vi "testCANopen.vi"() -> ()   [LabVIEW 2024]
doc: "Tests CANopen (and possibly CANbus) nets exercising the CANopen.lvclass APIs."
uses:
  CANopen/Multiplexor.ctl
  CANopen/FunctionCode.ctl
  DSP402/DSP402.lvclass
  CANopen/CANopen.lvclass
  DSP402/DriveState.ctl
  DSP402/DriveMode.ctl
  HAL/HAL/Devices/CAN Interfaces/PCAN/PCAN.lvclass
  D:/git/HAL/HAL/Configurations/CFG Base/CFG Base.lvclass
  D:/git/HAL/HAL/Protocols/ICAN/ICAN.lvclass
  CANopen/CANopen.lvclass/CANopen.ctl
  types/threestateFlag.ctl
  canopen.lvlib
  HAL/HAL/Configurations/CFG Base/CFG Base.lvclass
panel:
  in  "CANopen":refnum<class "CANopen.lvclass">
  in  "DSP402":refnum<class "DSP402.lvclass">
  in  "Variant":variant=variant(u8[] [80, 0])
  in  "Tab Control":T1(tab)
  in  "NMT send":bool
  in  "Node ID (NMT)":u8=50 caption="Node ID"
  in  "Command specifier":u8(ring)=129 items=["Start remote node"=1, "Stop remote node"=2, "Enter pre-operational state"=128, "Reset node"=129, "Reset communication"=130]
  in  "SDO size":u8=2 caption="Bytes" format="%0d"
  in  "SDO read":bool
  in  "Multiplexor":T2={"Index"=4119, "Sub-index"=0} {"Sub-index" format="%02x"; "Index" format="%04x"}
  in  "SDO value":u32 caption="Value" format="%08x"
  in  "SDO write":bool
  in  "Node ID (SDO)":u8=50 caption="Node ID"
  in  "Remap TxPDO":bool
  in  "TxPDO map":cluster{"CobID":u32, "nBytes":u8}[](array[cluster])=[{"CobID"=434, "nBytes"=2}] {"CobID" format="%x"}
  out "Input image":bool[](array[boolean])
  in  "Remap RxPDO":bool
  in  "RxPDO map":cluster{"CobID":u32, "nBytes":u8}[](array[cluster])=[{"CobID"=562, "nBytes"=5}] {"CobID" format="%x"}
  in  "Output image":bool[](array[boolean])
  in  "Node ID (402)":u8 caption="Node ID"
  in  "State (402)":T3 caption="State"
  in  "Mode (402)":T4 caption="Mode" items=["Undefined"=0, "Profile Position Mode"=1, "Velocity Mode"=2, "Profile Velocity Mode"=3, "Torque Profile Mode"=4, "Homing Mode"=6, "Interpolated Position Mode"=7]
  in  "Position (402)":u32 caption="Position"
  in  "Speed (402)":i16=500 caption="Speed (RpM)"
  in  "Operation flags (402)":cluster{"ON":bool, "OFF":bool}[](array[cluster]) caption="Force bit 4, 5, 6 and Halt"
  in  "Acceleration (402)":u32=100 caption="Acc"
  in  "Deceleration (402)":u32=100 caption="Dec"
  in  "Get status (402)":bool
  in  "PDO unlink":bool
  in  "PDO link":bool
  in  "Node ID (link)":u8=50 caption="Node ID"
  in  "Function code (link)":T5=4 caption="Function code" items=["NMT", "SYNC", "TIME STAMP", "EMERGENCY", "PDO1 (tx)", "PDO1 (rx)", "PDO2 (tx)", "PDO2 (rx)", "PDO3 (tx)", "PDO3 (rx)", "PDO4 (tx)", "PDO4 (rx)", "SDO (tx)", "SDO (rx)", "NMT Error Control"]
  in  "Indices":cluster{"Communication":u32, "Mapping":u32}={"Communication"=6144, "Mapping"=6656} {"Mapping" format="%x"; "Communication" format="%x"}
  in  "Map":cluster{"Multiplexor":T2, "nBits":u8}[](array[cluster])=[{"Multiplexor"={"Index"=24832, "Sub-index"=1}, "nBits"=16}] {"Multiplexor"."Sub-index" format="%02x"; "Multiplexor"."Index" format="%04x"}
  in  "Heartbeat set":bool
  in  "Heartbeat table":T6(array[cluster]) {"Period" format="%#.3g"}
  in  "Raw send":bool
  in  "Data (raw)":u8[](array[numeric]) caption="Data" format="%02x"
  in  "Node ID (raw)":u8 caption="Node ID"
  in  "Function code (raw)":T5=1 items=["NMT", "SYNC", "TIME STAMP", "EMERGENCY", "PDO1 (tx)", "PDO1 (rx)", "PDO2 (tx)", "PDO2 (rx)", "PDO3 (tx)", "PDO3 (rx)", "PDO4 (tx)", "PDO4 (rx)", "SDO (tx)", "SDO (rx)", "NMT Error Control"]
  in  "Stop":bool
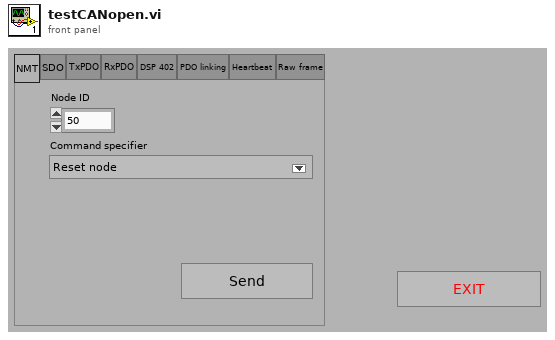
[diagram p1: front panel]
types:
  T1 = enum32{"NMT", "SDO", "TxPDO", "RxPDO", "DSP 402", "PDO linking", "Heartbeat", "Raw frame"}
  T2 = typedef "canopen.lvlib/CANopen.lvclass/Multiplexor.ctl" = cluster{"Index":u16, "Sub-index":u8}
  T3 = typedef "canopen.lvlib/DSP402.lvclass/DriveState.ctl" = enum16{"Start", "Not ready to switch on", "Switch on disabled", "Ready to switch on", "Switched on", "Operation enable", "Fault reaction active", "Fault", "Quick stop active"}
  T4 = typedef "canopen.lvlib/DSP402.lvclass/DriveMode.ctl" = i8
  T5 = typedef "canopen.lvlib/CANopen.lvclass/FunctionCode.ctl" = u8
  T6 = cluster{"Node ID":u8, "Period":dbl, "Set value":i16, "Value":i16}[]
  T7 = typedef "canopen.lvlib/threestateFlag.ctl" = i8
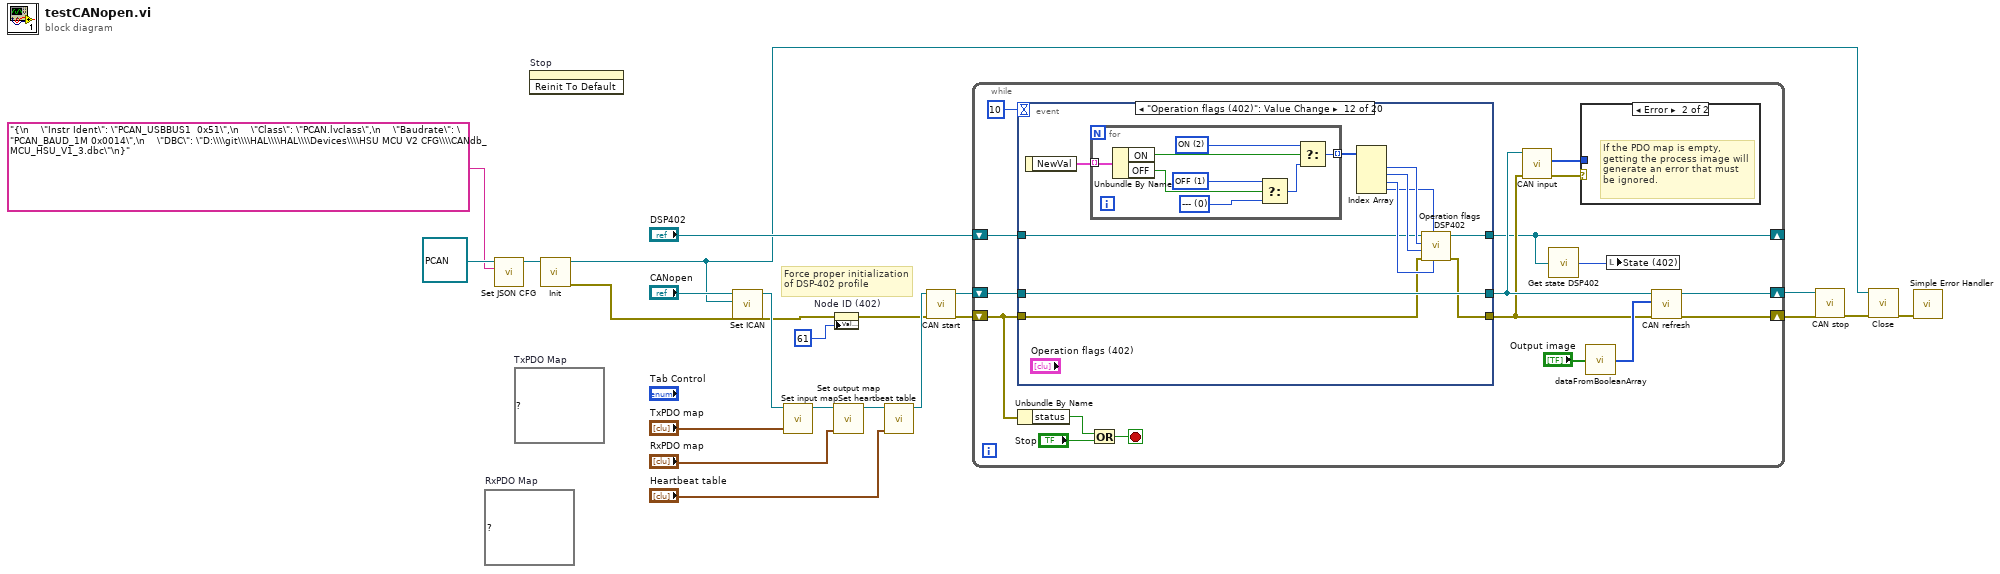
[diagram p0: block diagram]
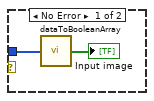
[diagram p2: hidden frame]
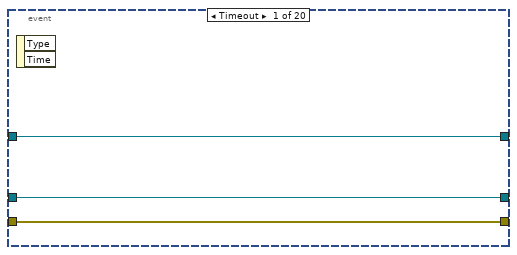
[diagram p3: hidden frame]
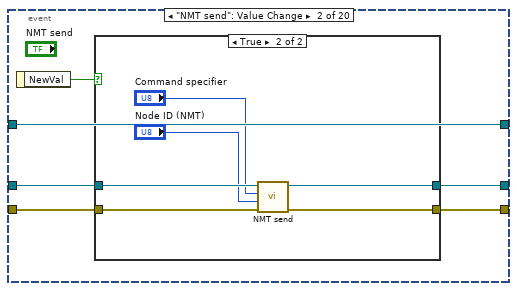
[diagram p4: hidden frame]
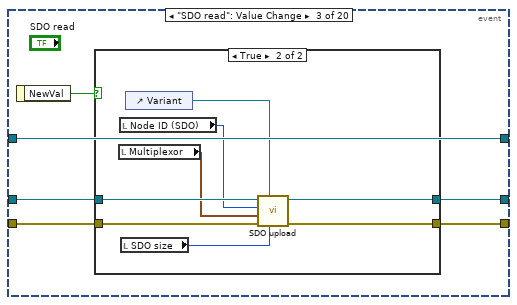
[diagram p6: hidden frame]
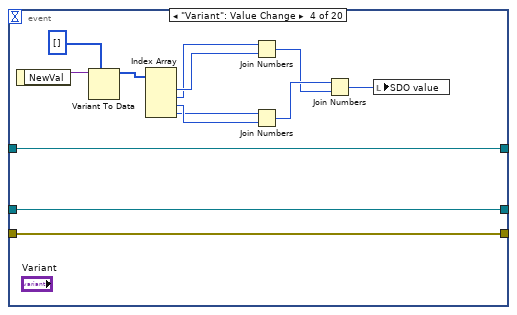
[diagram p8: hidden frame]
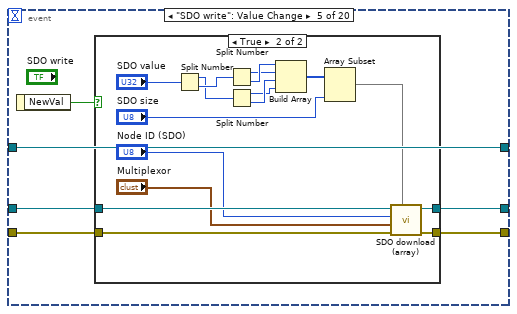
[diagram p9: hidden frame]
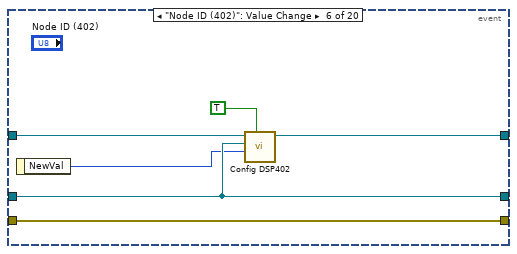
[diagram p11: hidden frame]
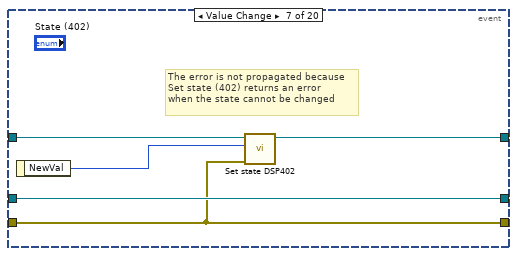
[diagram p12: hidden frame]
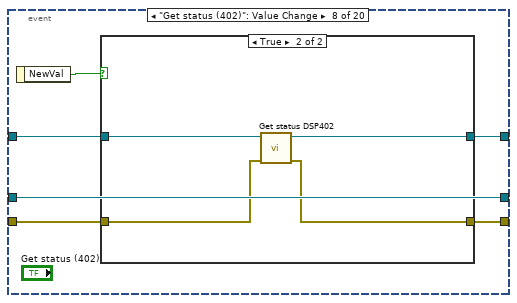
[diagram p13: hidden frame]
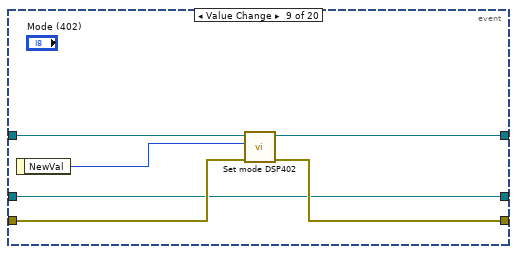
[diagram p15: hidden frame]
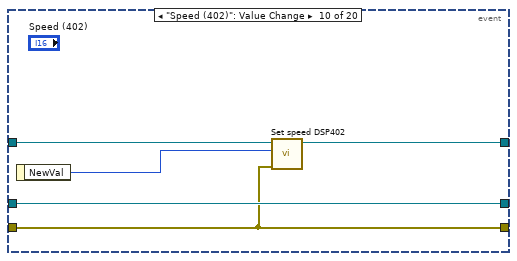
[diagram p16: hidden frame]
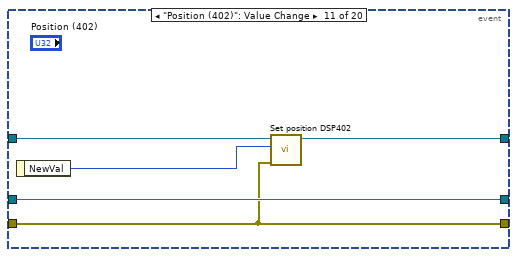
[diagram p17: hidden frame]
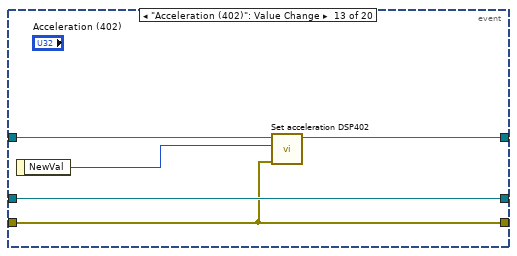
[diagram p18: hidden frame]
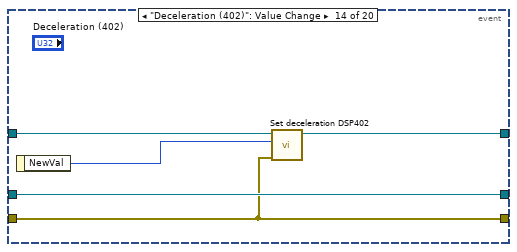
[diagram p19: hidden frame]
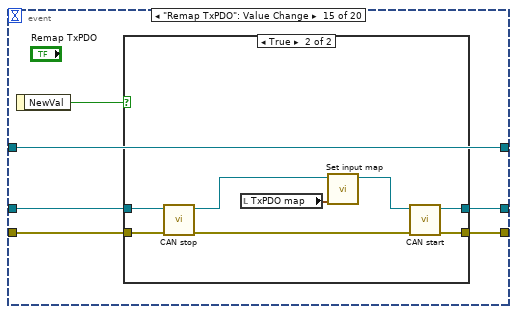
[diagram p20: hidden frame]
diagram:
  (unwired) map{u32, u32} {}  # RxPDO Map
  (unwired) map{u32, u32} {}  # TxPDO Map
  # "Force proper initialization\nof DSP-402 profile"
  n1 = call "Set JSON CFG.vi"("<JSON>CFG"="{\n    \"Instr Ident\": \"PCAN_USBBUS1  0x51\",\n    \"Class\": \"PCAN.lvclass\",\n    \"Baudrate\": \"PCAN_BAUD_1M 0x0014\",\n    \"DBC\": \"D:\\\\git\\\\HAL\\\\HAL\\\\Devices\\\\HSU MCU V2 CFG\\\\CANdb_MCU_HSU_V1_3.dbc\"\n}", "CFG Base in"=refnum<class "PCAN.lvclass"> refnum ("PCAN.lvclass")) -> ("CFG Base out"=w9:refnum<class "PCAN.lvclass">)  [unwired: 9 in]
  n2 = invoke on="Stop" class="Bool (strict)" method="Reinit To Default"() -> ()  [unwired: 3 in, 3 out]
  n3 = call-dynamic "Init.vi"("PCAN in"=w9) -> ("error out"=w1:errorcluster, "PCAN out"=w7:refnum<class "PCAN.lvclass">)  [unwired: 9 in]
  n4 = call "Set ICAN.vi"("ICAN"=w7, "CANopen in"="CANopen") -> ("CANopen out"=w2:refnum<class "CANopen.lvclass">)  [unwired: 9 in]
  n5 = call "Set input map.vi"("Map"="TxPDO map", "CANopen in"=w2) -> ("CANopen out"=w19:refnum<class "CANopen.lvclass">)  [unwired: 5 out]
  n6 = call "Set output map.vi"("Map"="RxPDO map", "CANopen in"=w19) -> ("CANopen out"=w17:refnum<class "CANopen.lvclass">)  [unwired: 5 out]
  n7 = property on="Node ID (402)" class="DigNum (strict)"(error in=w1, "Val(Sgnl)"=u8 61 ("Value (Signaling)")) -> (error out=w12:errorcluster)  [unwired: 1 in, 1 out]
  n8 = call "Set heartbeat table.vi"("Heartbeat table"="Heartbeat table", "CANopen in"=w17) -> ("CANopen out"=w15:refnum<class "CANopen.lvclass">)  [unwired: 1 in, 4 out]
  n9 = call "CAN start.vi"("error in (no error)"=w12, "CANopen in"=w15) -> ("error out"=w14:errorcluster, "CANopen out"=w20:refnum<class "CANopen.lvclass">)  [unwired: 4 out]
  n10 = while {
    shift-right: [w29] -> w5
    shift-left: w14 -> [w37]
    shift-right: [w28] -> w3
    shift-left: w20 -> [w39]
    shift-right: [w24] -> _
    shift-left: "DSP402" -> [w25]
    stop <- w36 stop-if-true
    n11 = event shown="[11] \"Operation flags (402)\": Value Change" {
      selector: _ -> [_ _ _ _ _ _ _ _ _ _ _ _ _ _ _ _ _ _ _ _]
      dyn-events: _ -> [_ _ _ _ _ _ _ _ _ _ _ _ _ _ _ _ _ _ _ _]
      timeout: 10 -> [_ _ _ _ _ _ _ _ _ _ _ _ _ _ _ _ _ _ _ _]
      tunnel: [w44 w50 w64 w87 w93 w115 w122 w123 w138 w145 w150 w160 w174 w179 w185 w201 w217 w229 w246 w262] -> w27
      tunnel: w39 -> [w44 w49 w63 w87 w92 w115 w122 w123 w138 w145 w150 w160 w174 w179 w184 w200 w216 w228 w245 w261]
      tunnel: [w43 w48 w62 w86 w91 w113 w118 w128 w139 w141 w146 w153 w170 w175 w183 w199 w215 w227 w244 w260] -> w26
      tunnel: w37 -> [w43 w47 w61 w86 w90 w113 w118 w127 w140 w141 w146 w154 w170 w175 w182 w198 w214 w226 w243 w259]
      tunnel: w25 -> [w42 w45 w59 w75 w88 w117 w120 w124 w136 w143 w149 w151 w172 w177 w180 w196 w212 w224 w241 w257]
      tunnel: [w42 w45 w59 w75 w88 w116 w119 w125 w135 w142 w148 w152 w171 w176 w180 w196 w212 w224 w241 w257] -> w24
      event Timeout {
        n12 = event-data() -> ()  [unwired: 3 out]
      }
      event "NMT send": Value Change {
        n13 = event-data() -> ("NewVal"=w46:bool)  [unwired: 1 out]
        n14 = case shown="True" w46 {
          tunnel: [w52 w55] -> w50
          tunnel: w49 -> [w52 w58]
          tunnel: [w51 w56] -> w48
          tunnel: w47 -> [w51 w57]
          frame False {
          }
          frame True {
            n15 = call "NMT send.vi"("error in (no error)"=w57, "Node ID"="Node ID (NMT)", "Command specifier"="Command specifier", "CANopen in"=w58) -> ("error out"=w56:errorcluster, "CANopen out"=w55:refnum<class "CANopen.lvclass">)  [unwired: 1 in, 1 out]
          }
        }
      }
      event "SDO read": Value Change {
        n16 = event-data() -> ("NewVal"=w60:bool)  [unwired: 1 out]
        n17 = case shown="True" w60 {
          tunnel: [w66 w71] -> w64
          tunnel: w63 -> [w66 w74]
          tunnel: [w65 w72] -> w62
          tunnel: w61 -> [w65 w73]
          frame False {
          }
          frame True {
            n18 = local read "Multiplexor"() -> (w69:T2)
            n19 = local read "Node ID (SDO)"() -> (w70:u8)
            n20 = local read "SDO size"() -> (w67:u8)
            n21 = control-ref of="Variant"() -> (w68:refnum<vi>)
            n22 = call "SDO upload.vi"("Size"=w67, "Destination"=w68, "error in (no error)"=w73, "Multiplexor"=w69, "Node ID"=w70, "CANopen in"=w74) -> ("error out"=w72:errorcluster, "CANopen out"=w71:refnum<class "CANopen.lvclass">)  [unwired: 2 out]
          }
        }
      }
      event "Variant": Value Change {
        n23 = event-data() -> ("NewVal"=w84:variant)  [unwired: 1 out]
        n24 = Variant To Data(type=u8[] [] ("Data"), Variant=w84) -> (data=w82:u8[])  [unwired: 1 in, 1 out]
        n25 = Index Array(array=w82) -> (element #1=w81:u8, element #2=w80:u8, element #3=w79:u8, element #4=w78:u8)  [unwired: 4 in]
        n26 = Join Numbers(hi=w80, lo=w81) -> ((hi.lo)=w76:u16)
        n27 = Join Numbers(hi=w78, lo=w79) -> ((hi.lo)=w77:u16)
        n28 = Join Numbers(hi=w77, lo=w76) -> ((hi.lo)=w83:u32)
        n29 = local write "SDO value"(w83) -> ()
      }
      event "SDO write": Value Change {
        n30 = event-data() -> ("NewVal"=w89:bool)  [unwired: 1 out]
        n31 = case shown="True" w89 {
          tunnel: [w95 w108] -> w93
          tunnel: w92 -> [w95 w111]
          tunnel: [w94 w109] -> w91
          tunnel: w90 -> [w94 w110]
          frame False {
          }
          frame True {
            n32 = Split Number(x="SDO value") -> (hi(x)=w102:u16, lo(x)=w104:u16)
            n33 = Split Number(x=w104) -> (hi(x)=w101:u8, lo(x)=w103:u8)
            n34 = Split Number(x=w102) -> (hi(x)=w99:u8, lo(x)=w100:u8)
            n35 = Build Array(w103, w101, w100, w99) -> (w98:u8[])
            n36 = Array Subset(array=w98, length="SDO size") -> (w96:u8[])  [unwired: 1 in]
            n37 = call "SDO download (array).vi"("Value"=w96, "error in (no error)"=w110, "Multiplexor"="Multiplexor", "Node ID"="Node ID (SDO)", "CANopen in"=w111) -> ("error out"=w109:errorcluster, "CANopen out"=w108:refnum<class "CANopen.lvclass">)  [unwired: 1 in, 2 out]
          }
        }
      }
      event "Node ID (402)": Value Change {
        n38 = event-data() -> ("NewVal"=w114:u8)  [unwired: 1 out]
        n39 = call "Config DSP402.vi"("Wait?"=TRUE, "Node ID"=w114, "CANopen"=w115, "DSP402 in"=w117) -> ("DSP402 out"=w116:refnum<class "DSP402.lvclass">)  [unwired: 1 in, 4 out]
      }
      event Value Change {
        # "The error is not propagated because\nSet state (402) returns an error\nwhen the state cannot be changed"
        n40 = event-data() -> ("NewVal"=w121:T3)  [unwired: 1 out]
        n41 = call "Set state DSP402.vi"("error in (no error)"=w118, "State"=w121, "DSP402 in"=w120) -> ("DSP402 out"=w119:refnum<class "DSP402.lvclass">)  [unwired: 4 out]
      }
      event "Get status (402)": Value Change {
        n42 = event-data() -> ("NewVal"=w126:bool)  [unwired: 1 out]
        n43 = case shown="True" w126 {
          tunnel: [w130 w133] -> w128
          tunnel: w127 -> [w130 w134]
          tunnel: [w129 w131] -> w125
          tunnel: w124 -> [w129 w132]
          frame False {
          }
          frame True {
            n44 = call "Get status DSP402.vi"("error in (no error)"=w134, "DSP402 in"=w132) -> ("error out"=w133:errorcluster, "DSP402 out"=w131:refnum<class "DSP402.lvclass">)  [unwired: 1 in, 3 out]
          }
        }
      }
      event Value Change {
        n45 = event-data() -> ("NewVal"=w137:T4)  [unwired: 1 out]
        n46 = call "Set mode DSP402.vi"("error in (no error)"=w140, "Mode"=w137, "DSP402 in"=w136) -> ("error out"=w139:errorcluster, "DSP402 out"=w135:refnum<class "DSP402.lvclass">)  [unwired: 3 out]
      }
      event "Speed (402)": Value Change {
        n47 = event-data() -> ("NewVal"=w144:i16)  [unwired: 1 out]
        n48 = call "Set speed DSP402.vi"("error in (no error)"=w141, "RpM"=w144, "DSP402 in"=w143) -> ("DSP402 out"=w142:refnum<class "DSP402.lvclass">)  [unwired: 8 out]
      }
      event "Position (402)": Value Change {
        n49 = event-data() -> ("NewVal"=w147:u32)  [unwired: 1 out]
        n50 = call "Set position DSP402.vi"("error in (no error)"=w146, "Position units"=w147, "DSP402 in"=w149) -> ("DSP402 out"=w148:refnum<class "DSP402.lvclass">)  [unwired: 3 in, 5 out]
      }
      event "Operation flags (402)": Value Change {
        n51 = event-data() -> ("NewVal"=w161:cluster{"ON":bool, "OFF":bool}[])  [unwired: 1 out]
        n52 = for {
          tunnel: w161 -> [w169] mode=indexing
          tunnel: [w163] -> w159 mode=indexing
          w167 = T7 2 items=["---", "OFF", "ON"] ("Flag")
          w164 = T7 1 items=["---", "OFF", "ON"] ("Flag")
          w162 = T7 0 items=["---", "OFF", "ON"] ("Flag")
          n53 = Unbundle By Name(w169) -> ("ON"=w168:bool, "OFF"=w166:bool)
          n54 = Select(t=w164, s=w166, f=w162) -> (s? t:f=w165:T7)
          n55 = Select(t=w167, s=w168, f=w165) -> (s? t:f=w163:T7)
        }
        n56 = Index Array(array=w159) -> (element #1=w158:T7, element #2=w157:T7, element #3=w156:T7, element #4=w155:T7)  [unwired: 4 in]
        n57 = call "Operation flags DSP402.vi"("Bit 6"=w156, "Halt"=w155, "error in (no error)"=w154, "Bit 5"=w157, "Bit 4"=w158, "DSP402 in"=w151) -> ("error out"=w153:errorcluster, "DSP402 out"=w152:refnum<class "DSP402.lvclass">)  [unwired: 4 out]
      }
      event "Acceleration (402)": Value Change {
        n58 = event-data() -> ("NewVal"=w173:u32)  [unwired: 1 out]
        n59 = call "Set acceleration DSP402.vi"("error in (no error)"=w170, "Acceleration units"=w173, "DSP402 in"=w172) -> ("DSP402 out"=w171:refnum<class "DSP402.lvclass">)  [unwired: 8 out]
      }
      event "Deceleration (402)": Value Change {
        n60 = event-data() -> ("NewVal"=w178:u32)  [unwired: 1 out]
        n61 = call "Set deceleration DSP402.vi"("error in (no error)"=w175, "Deceleration units"=w178, "DSP402 in"=w177) -> ("DSP402 out"=w176:refnum<class "DSP402.lvclass">)  [unwired: 8 out]
      }
      event "Remap TxPDO": Value Change {
        n62 = event-data() -> ("NewVal"=w181:bool)  [unwired: 1 out]
        n63 = case shown="True" w181 {
          tunnel: [w187 w194] -> w185
          tunnel: w184 -> [w187 w189]
          tunnel: [w186 w195] -> w183
          tunnel: w182 -> [w186 w192]
          frame False {
          }
          frame True {
            n64 = call "CAN stop.vi"("error in (no error)"=w192, "CANopen in"=w189) -> ("error out"=w191:errorcluster, "CANopen out"=w188:refnum<class "CANopen.lvclass">)  [unwired: 4 out]
            n65 = local read "TxPDO map"() -> (w190:cluster{"CobID":u32, "nBytes":u8}[])
            n66 = call "Set input map.vi"("Map"=w190, "CANopen in"=w188) -> ("CANopen out"=w193:refnum<class "CANopen.lvclass">)  [unwired: 5 out]
            n67 = call "CAN start.vi"("error in (no error)"=w191, "CANopen in"=w193) -> ("error out"=w195:errorcluster, "CANopen out"=w194:refnum<class "CANopen.lvclass">)  [unwired: 4 out]
          }
        }
      }
      event "Heartbeat set": Value Change {
        n68 = event-data() -> ("NewVal"=w197:bool)  [unwired: 1 out]
        n69 = case shown="True" w197 {
          tunnel: [w203 w210] -> w201
          tunnel: w200 -> [w203 w205]
          tunnel: [w202 w211] -> w199
          tunnel: w198 -> [w202 w208]
          frame False {
          }
          frame True {
            n70 = call "CAN stop.vi"("error in (no error)"=w208, "CANopen in"=w205) -> ("error out"=w207:errorcluster, "CANopen out"=w204:refnum<class "CANopen.lvclass">)  [unwired: 4 out]
            n71 = local read "Heartbeat table"() -> (w206:T6)
            n72 = call "Set heartbeat table.vi"("Heartbeat table"=w206, "CANopen in"=w204) -> ("CANopen out"=w209:refnum<class "CANopen.lvclass">)  [unwired: 5 out]
            n73 = call "CAN start.vi"("error in (no error)"=w207, "CANopen in"=w209) -> ("error out"=w211:errorcluster, "CANopen out"=w210:refnum<class "CANopen.lvclass">)  [unwired: 4 out]
          }
        }
      }
      event "Remap RxPDO": Value Change {
        n74 = event-data() -> ("NewVal"=w213:bool)  [unwired: 1 out]
        n75 = case shown="True" w213 {
          tunnel: [w219 w220] -> w217
          tunnel: w216 -> [w219 w222]
          tunnel: [w218 w221] -> w215
          tunnel: w214 -> [w218 w221]
          frame False {
          }
          frame True {
            n76 = local read "RxPDO map"() -> (w223:cluster{"CobID":u32, "nBytes":u8}[])
            n77 = call "Set output map.vi"("Map"=w223, "CANopen in"=w222) -> ("CANopen out"=w220:refnum<class "CANopen.lvclass">)  [unwired: 5 out]
          }
        }
      }
      event "PDO link": Value Change {
        n78 = event-data() -> ("NewVal"=w225:bool)  [unwired: 1 out]
        n79 = case shown="True" w225 {
          tunnel: [w231 w237] -> w229
          tunnel: w228 -> [w231 w240]
          tunnel: [w230 w238] -> w227
          tunnel: w226 -> [w230 w239]
          frame False {
          }
          frame True {
            n80 = call "enCOB-ID.vi"("Function code"="Function code (link)", "Node ID"="Node ID (link)") -> ("Cob ID"=w235:u32)
            n81 = call "PDO link.vi"("Map"="Map", "error in (no error)"=w239, "Indices"="Indices", "Cob ID"=w235, "CANopen in"=w240) -> ("error out"=w238:errorcluster, "CANopen out"=w237:refnum<class "CANopen.lvclass">)  [unwired: 1 in, 2 out]
          }
        }
      }
      event "PDO unlink": Value Change {
        n82 = event-data() -> ("NewVal"=w242:bool)  [unwired: 1 out]
        n83 = case shown="True" w242 {
          tunnel: [w248 w253] -> w246
          tunnel: w245 -> [w248 w256]
          tunnel: [w247 w254] -> w244
          tunnel: w243 -> [w247 w255]
          frame False {
          }
          frame True {
            n84 = local read "Function code (link)"() -> (w250:T5)
            n85 = local read "Node ID (link)"() -> (w251:u8)
            n86 = local read "Indices"() -> (w249:cluster{"Communication":u32, "Mapping":u32})
            n87 = call "enCOB-ID.vi"("Function code"=w250, "Node ID"=w251) -> ("Cob ID"=w252:u32)
            n88 = call "PDO unlink.vi"("error in (no error)"=w255, "Indices"=w249, "Cob ID"=w252, "CANopen in"=w256) -> ("error out"=w254:errorcluster, "CANopen out"=w253:refnum<class "CANopen.lvclass">)  [unwired: 1 in, 2 out]
          }
        }
      }
      event "Raw send": Value Change {
        n89 = event-data() -> ("NewVal"=w258:bool)  [unwired: 1 out]
        n90 = case shown="True" w258 {
          tunnel: [w264 w269] -> w262
          tunnel: w261 -> [w264 w272]
          tunnel: [w263 w270] -> w260
          tunnel: w259 -> [w263 w271]
          frame False {
          }
          frame True {
            n91 = call "enCOB-ID.vi"("Function code"="Function code (raw)", "Node ID"="Node ID (raw)") -> ("Cob ID"=w267:u32)
            n92 = call "CAN write.vi"("error in (no error)"=w271, "Data"="Data (raw)", "COB id"=w267, "CANopen in"=w272) -> ("error out"=w270:errorcluster, "CANopen out"=w269:refnum<class "CANopen.lvclass">)  [unwired: 1 in, 1 out]
          }
        }
      }
    }
    n93 = Unbundle By Name(w37) -> ("status"=w34:bool)
    n94 = Or(x=w34, y="Stop") -> (x .or. y?=w36:bool)
    n95 = call "CAN input.vi"("error in (no error)"=w26, "CANopen"=w27) -> ("error out"=w33:errorcluster, "Input image"=w32:u8[])  [unwired: 8 out]
    n96 = call-dynamic "Get state DSP402.vi"("DSP402 in"=w24) -> ("State"=w23:T3)
    n97 = case shown="Error" w33 {
      tunnel: w32 -> [w40 _]
      frame No Error {
        n98 = call "dataToBooleanArray.vi"("Data"=w40) -> ("Boolean array"=→"Input image":bool[])
      }
      frame Error {
        # "If the PDO map is empty,\ngetting the process image will\ngenerate an error that must\nbe ignored."
      }
    }
    n99 = call "dataFromBooleanArray.vi"("Boolean array"="Output image") -> ("Data"=w30:u8[])
    n100 = local write "State (402)"(w23) -> ()
    n101 = call "CAN refresh.vi"("error in (no error)"=w26, "Output image"=w30, "CANopen in"=w27) -> ("error out"=w29:errorcluster, "CANopen out"=w28:refnum<class "CANopen.lvclass">)  [unwired: 1 in, 2 out]
  }
  n102 = call "CAN stop.vi"("error in (no error)"=w5, "CANopen in"=w3) -> ("error out"=w4:errorcluster)  [unwired: 4 in, 1 out]
  n103 = call-dynamic "Close.vi"("error in"=w4, "PCAN in"=w7) -> ("error out"=w6:errorcluster)  [unwired: 8 in, 1 out]
  n104 = call <vilib>:"Simple Error Handler.vi"("error in (no error)"=w6) -> ()  [unwired: 1 in, 8 out]
